vi "Create Process from File.vi"(8 "error in (no error)":errorcluster, 10 "Process":path, 11 "Process Model in":refnum<class "Process Model.lvclass">) -> (0 "error out":errorcluster, 3 "Process Model out":refnum<class "Process Model.lvclass">)   [LabVIEW 2017, in "Car Wash.lvlib" / "Process Model.lvlib" / "Process Model.lvclass"]
uses:
  Process Model.lvclass
  <vilib>/gpm_packages/@cs/test-executive/Source/Test Executive/TestExecutive/Test Executive.lvclass
  C:/Program Files/National Instruments/LabVIEW 2017/user.lib/composed/test-executive/Source/Test Executive/ITestExecutive/ITest Executive.lvclass
  <vilib>/gpm_packages/@cs/persistence/source/XML/XML.lvclass
  C:/Program Files/National Instruments/LabVIEW 2017/user.lib/composed/persistence/source/IPersist/IPersist.lvclass
  Process Model.lvclass/Process Model.ctl
  <vilib>/gpm_packages/@cs/test-executive/Source/Test Executive/TestExecutive Ref/TestExecutive Ref.lvclass
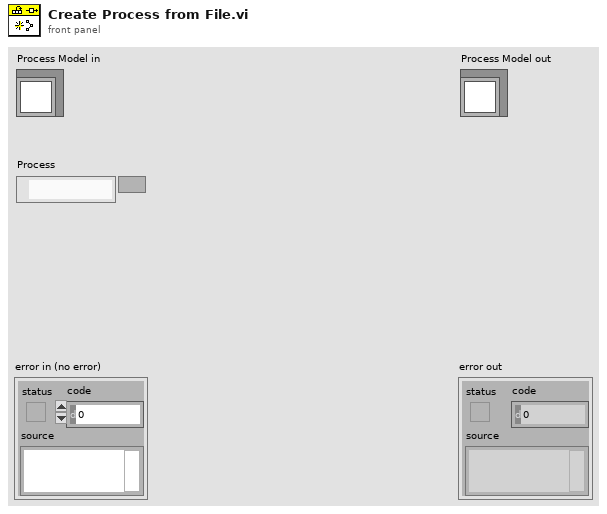
[diagram p1: front panel]
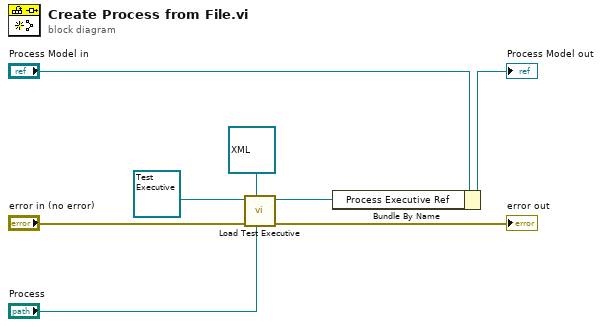
[diagram p0: block diagram]
diagram:
  n1 = call <vilib>:"Load Test Executive.vi"("Folder"="Process", "Persistence in"=refnum<class "XML.lvclass"> refnum ("XML.lvlib:XML.lvclass"), "error in (no error)"="error in (no error)", "Test Executive"=refnum<class "Test Executive.lvclass"> refnum ("Test Executive.lvlib:Test Executive.lvclass")) -> ("error out"=→"error out":errorcluster, "Test Executive Ref out"=w4:refnum<data-value>)  [unwired: 5 in, 1 out]
  n2 = Bundle By Name(cluster="Process Model in", "Process Executive Ref"=w4) -> (→"Process Model out":refnum<class "Process Model.lvclass">)
